vi "sv_Prepare STFT blocks.vi"(0 "scaled signal [EU]":waveform(dbl), 1 "FFT info":T1={"FFT block size"=1024, "number of FFT"=0, "start index"=0, "increment"=0.0} {"increment" format="%.2f"}, 11 "error in (no error)":errorcluster, 12 "iteration":i32) -> (4 "scaled signal [EU]":waveform(dbl), 15 "error out":errorcluster)   [LabVIEW 2017, in "SoundVib_Transient.lvlib"]
uses:
  <vilib>/addons/Sound and Vibration/svt_Transients/SoundVib_Transient.lvlib
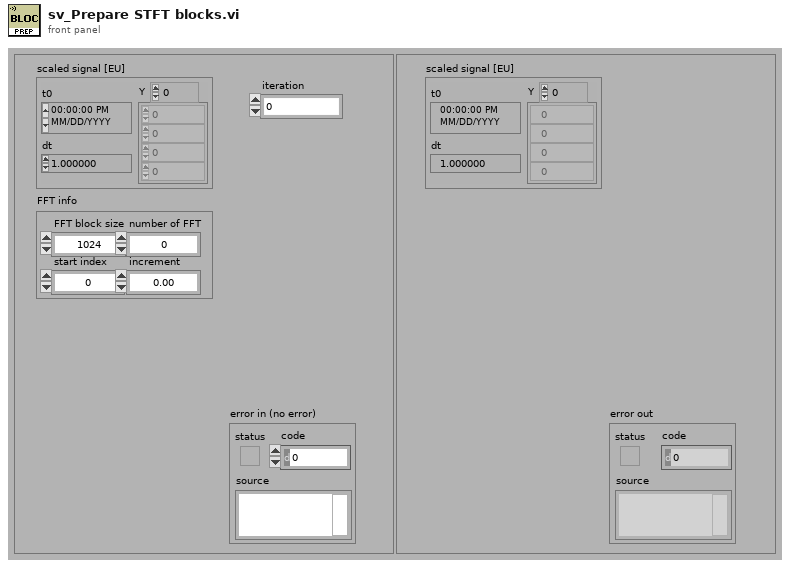
[diagram p1: front panel]
types:
  T1 = cluster{"FFT block size":i32, "number of FFT":i32, "start index":i32, "increment":dbl}
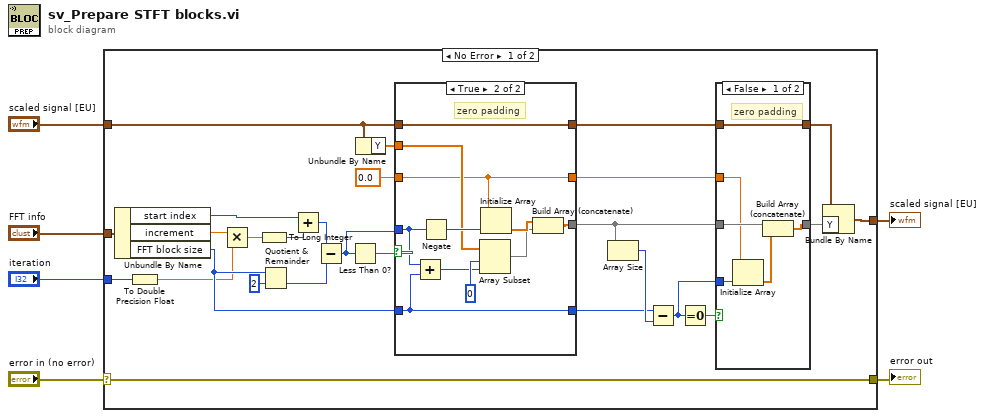
[diagram p0: block diagram]
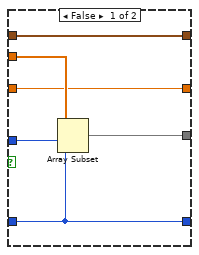
[diagram p2: hidden frame]
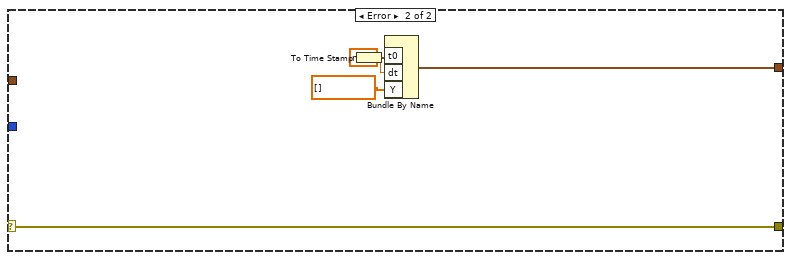
[diagram p4: hidden frame]
diagram:
  n1 = case shown="No Error" "error in (no error)" {
    selector: "error in (no error)" -> [w9 w63]
    tunnel: "scaled signal [EU]" -> [w14 _]
    tunnel: "FFT info" -> [w22 _]
    tunnel: [w10 w60] -> w3
    tunnel: [w9 w63] -> w2
    tunnel: "iteration" -> [w8 _]
    frame No Error {
      n2 = Unbundle By Name(w22) -> ("start index"=w21:i32, "increment"=w20:dbl, "FFT block size"=w17:i32)
      n3 = To Double Precision Float(number=w8) -> (double precision float=w7:dbl)
      n4 = Multiply(x=w20, y=w7) -> (x*y=w25:dbl)
      n5 = To Long Integer(number=w25) -> (32bit integer=w26:i32)
      n6 = Quotient & Remainder(x=w17, y=2) -> (floor(x/y)=w19:i32)  [unwired: 1 out]
      n7 = Add(x=w21, y=w26) -> (x+y=w27:i32)
      n8 = Subtract(x=w27, y=w19) -> (x-y=w16:i32)
      n9 = Less Than 0?(x=w16) -> (x < 0?=w30:bool)
      n10 = Unbundle By Name(w14) -> ("Y"=w23:dbl[])
      n11 = case shown="True" w30 {
        tunnel: w23 -> [w39 w49]
        tunnel: w17 -> [w37 w43]
        tunnel: [w38 w44] -> w28
        tunnel: [w37 w43] -> w18
        tunnel: w16 -> [w36 w42]
        tunnel: w14 -> [w35 w41]
        tunnel: [w35 w41] -> w15
        tunnel: 0.0 -> [w34 w40]
        tunnel: [w34 w40] -> w11
        frame False {
          n12 = Array Subset(array=w39, index=w36, length=w37) -> (w38:dbl[])
        }
        frame True {
          # "zero padding"
          n13 = Add(x=w42, y=w43) -> (x+y=w47:i32)
          n14 = Negate(x=w42) -> (-x=w50:i32)
          n15 = Array Subset(array=w49, index=0, length=w47) -> (w45:dbl[])
          n16 = Initialize Array(w40, w50) -> (w46:dbl[])
          n17 = Build Array (concatenate)(w46, w45) -> (w44:dbl[])
        }
      }
      n18 = Array Size(array=w28) -> (size(s)=w31:i32)
      n19 = Subtract(x=w18, y=w31) -> (x-y=w29:i32)
      n20 = Equal To 0?(x=w29) -> (x = 0?=w32:bool)
      n21 = case shown="False" w32 {
        tunnel: [w53 w58] -> w33
        tunnel: w28 -> [w56 w58]
        tunnel: w29 -> [w55 _]
        tunnel: w15 -> [w52 w57]
        tunnel: [w52 w57] -> w13
        tunnel: w11 -> [w51 _]
        frame False {
          # "zero padding"
          n22 = Initialize Array(w51, w55) -> (w54:dbl[])
          n23 = Build Array (concatenate)(w56, w54) -> (w53:dbl[])
        }
        frame True {
        }
      }
      n24 = Bundle By Name(cluster=w13, "Y"=w33) -> (w10:waveform(dbl))
    }
    frame Error {
      w62 = nan ("t0")
      n25 = To Time Stamp(1:w62) -> (0:w59:timestamp)
      n26 = Bundle By Name("t0"=w59, "dt"=w62, "Y"=dbl[] []) -> (w60:waveform(dbl))  [unwired: 1 in]
    }
  }
  "scaled signal [EU]" <- w3
  "error out" <- w2
